vi "CloneClass.vi"(0 "ClassWriterGOOP300.lvclass":refnum<class "ClassWriterGOOP300.lvclass">, 1 "ClassRef":refnum<vi>, 2 "NewClassPath":path, 5 "error in (no error)":errorcluster) -> (14 "ClassWriterGOOP300.lvclass":refnum<class "ClassWriterGOOP300.lvclass">, 16 "NewClassPathOut(Might Be Modified)":path, 19 "error out":errorcluster)   [LabVIEW 2020, in "ClassWriterGOOP300.lvclass"]
uses:
  ClassWriterGOOP300.lvclass
  Provider_LvNativeClass/ClassWriterNative_class/ClassWriterNative.lvclass
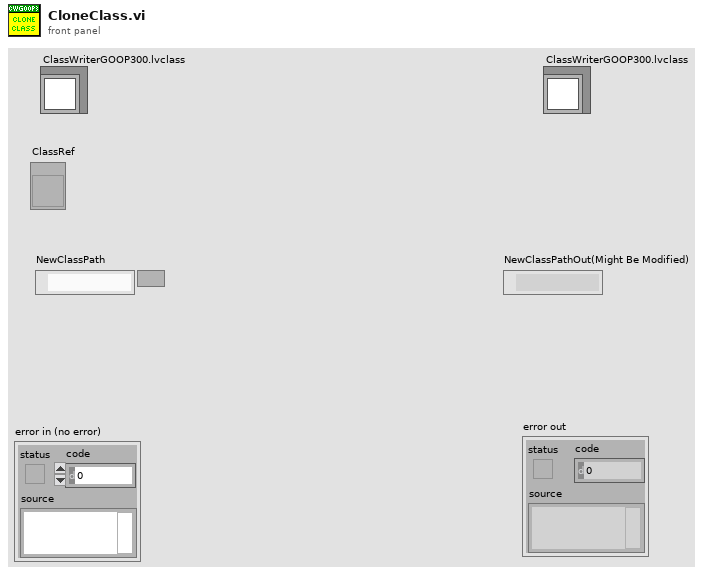
[diagram p1: front panel]
types:
  T1 = typedef "imagedata.ctl" = cluster{"image type":i32, "image depth":i32, "image":u8[], "mask":u8[], "colors":u32[], "Rectangle":cluster{"left":i16, "top":i16, "right":i16, "bottom":i16}}
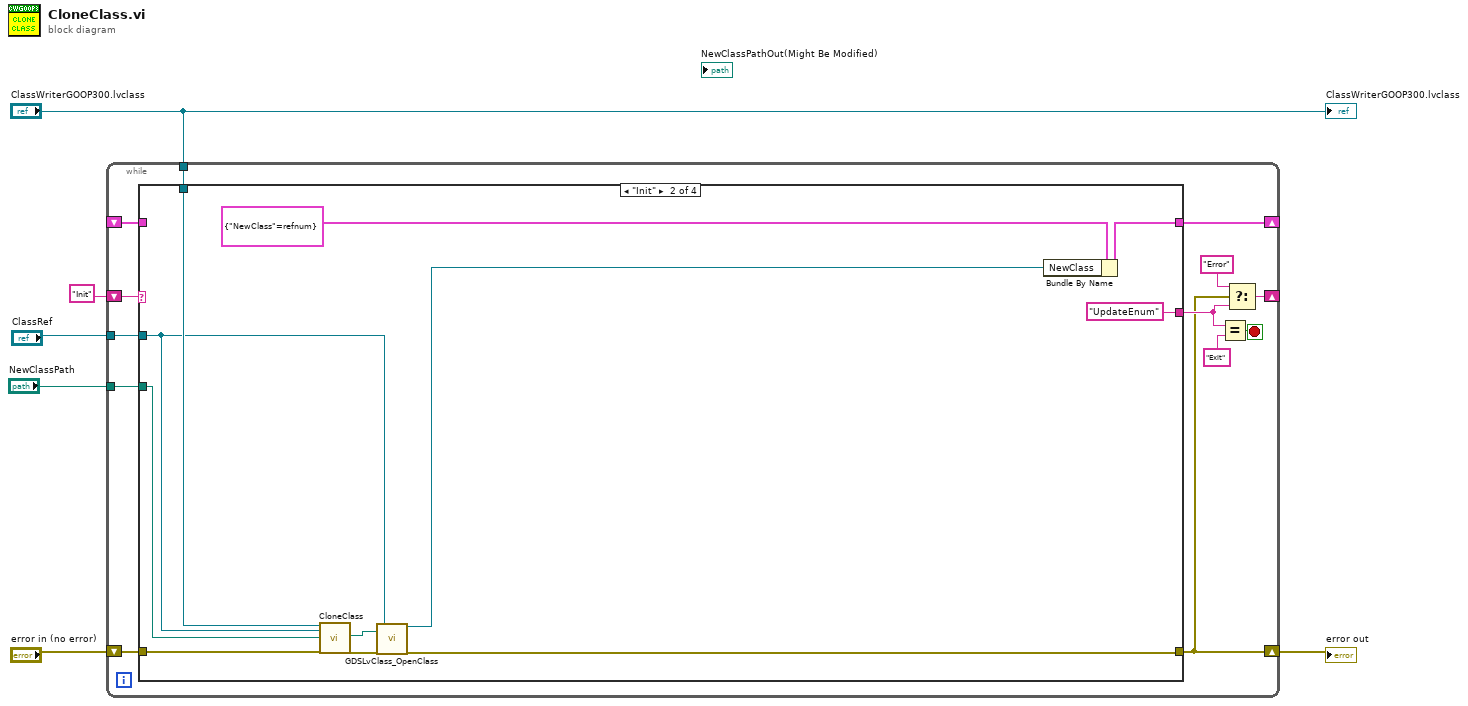
[diagram p0: block diagram]
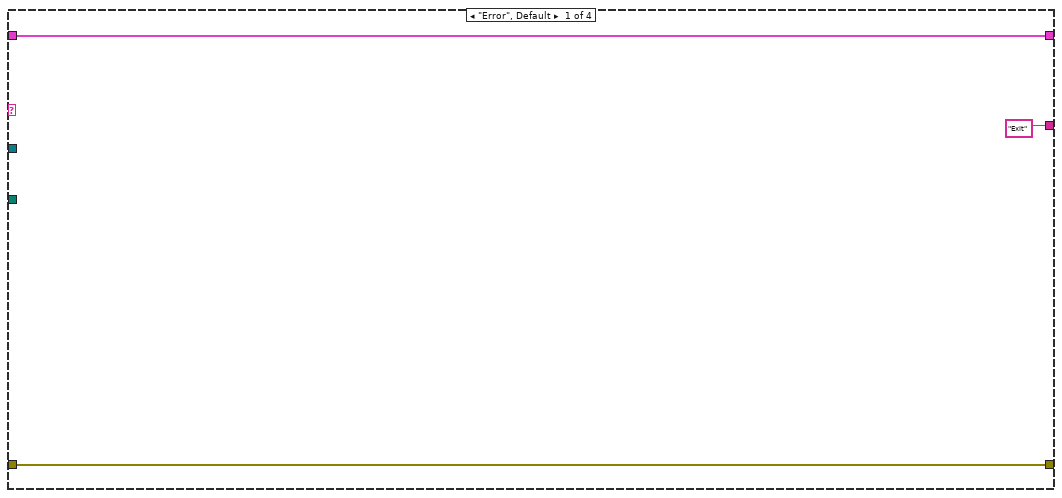
[diagram p2: hidden frame]
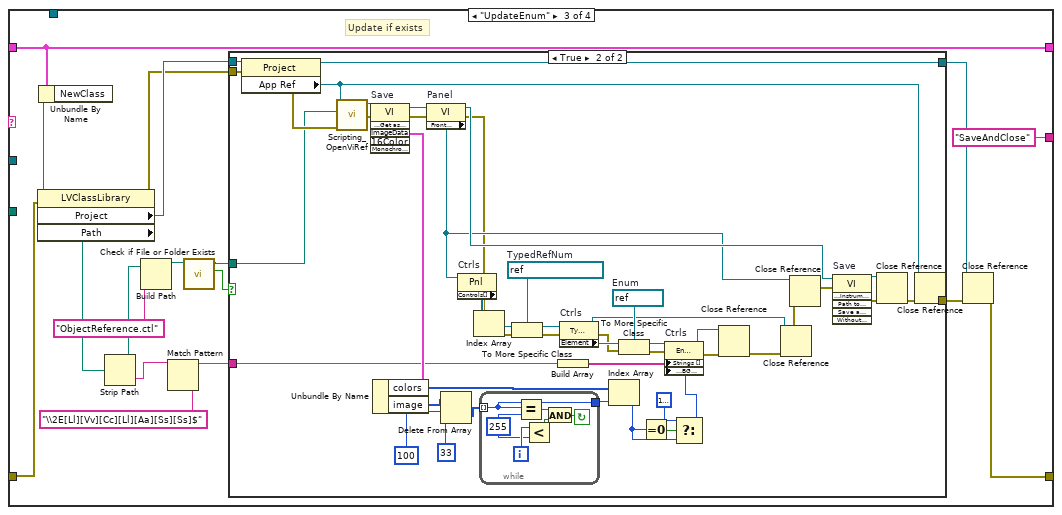
[diagram p3: hidden frame]
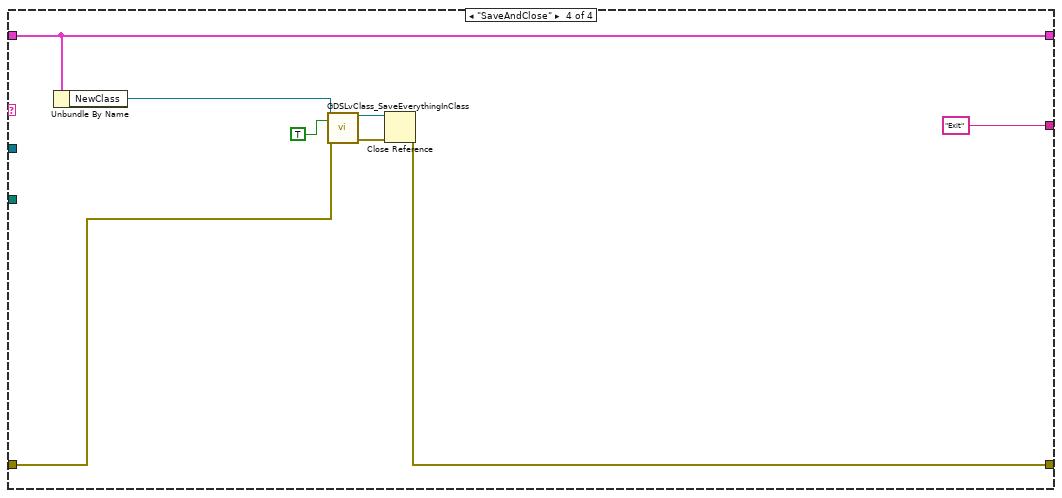
[diagram p5: hidden frame]
diagram:
  n1 = while {
    shift-right: [w12] -> w2
    shift-left: "error in (no error)" -> [w19]
    shift-right: [w17] -> _
    shift-left: "Init" -> [w18]
    shift-right: [w11] -> _
    shift-left: _ -> [w10]
    tunnel: "ClassWriterGOOP300.lvclass" -> [w9]
    tunnel: "ClassRef" -> [w8]
    tunnel: "NewClassPath" -> [w7]
    stop <- w16 stop-if-true
    n2 = case shown="\"Init\"" w18 {
      tunnel: w19 -> [w22 w30 w40 w108]
      tunnel: [w22 w26 w42 w111] -> w12
      tunnel: ["Exit" "UpdateEnum" "SaveAndClose" "Exit"] -> w13
      tunnel: [w20 w31 w50 w112] -> w11
      tunnel: w10 -> [w20 _ w50 w112]
      tunnel: w9 -> [_ w29 _ _]
      tunnel: w8 -> [_ w25 _ _]
      tunnel: w7 -> [_ w24 _ _]
      frame "Error", Default {
      }
      frame "Init" {
        n3 = call-parent "CloneClass.vi"("ClassWriterNative.lvclass"=w29, "ClassRef"=w25, "NewClassPath"=w24, "error in (no error)"=w30) -> ("NewClassPathOut(Might Be Modified)"=w23:path, "error out"=w28:errorcluster)  [unwired: 13 in, 1 out]
        n4 = call "GDSLvClass_OpenClass.vi"("ClassToOpen"=w23, "error in (no error)"=w28, "Project/ApplicationRef(If empty, currect active project will be used)"=w25) -> ("LVClass.Open"=w27:refnum<vi>, "error out"=w26:errorcluster)  [unwired: 15 in]
        n5 = Bundle By Name(cluster=cluster{"NewClass":refnum<vi>} {"NewClass"=refnum}, "NewClass"=w27) -> (w31:cluster{"NewClass":refnum<vi>})
      }
      frame "UpdateEnum" {
        # "Update if exists"
        n6 = Unbundle By Name(w50) -> ("NewClass"=w48:refnum<vi>)
        n7 = property class="LVClassLibrary"(reference=w48, error in=w40) -> (error out=w41:errorcluster, "Project"=w47:refnum<vi>, "Path"=w46:path)  [unwired: 1 out]
        n8 = Strip Path(path=w46) -> (stripped path=w45:path, name=w38:string)
        n9 = Build Path(base path=w45, name or relative path="ObjectReference.ctl") -> (appended path=w36:path)
        n10 = Match Pattern(string=w38, regular expression="\\2E[Ll][Vv][Cc][Ll][Aa][Ss][Ss]$") -> (before substring=w39:string)  [unwired: 1 in, 3 out]
        n11 = call <vilib>:"Check if File or Folder Exists.vi"("path"=w36) -> ("file or folder exists?"=w34:bool, "dup path"=w35:path)  [unwired: 8 in, 1 out]
        n12 = case shown="True" w34 {
          tunnel: w47 -> [w52 w59]
          tunnel: [w53 w58] -> w44
          tunnel: [w52 w57] -> w43
          tunnel: w41 -> [w53 w56]
          tunnel: w39 -> [_ w55]
          tunnel: w35 -> [_ w54]
          frame False {
          }
          frame True {
            w94 = refnum<vi> refnum  # Enum
            w97 = refnum<vi> refnum  # TypedRefNum
            n13 = property class="Project"(reference=w59, error in=w56) -> (reference out=w57:refnum<vi>, error out=w66:errorcluster, "App Ref"=w60:refnum<vi>)
            n14 = call "Scripting_OpenViRef.vi"("error in"=w66, "ViPath/ViName/Viref"=w54, "AppRef"=w60) -> ("error out"=w78:errorcluster, "vi reference"=w79:refnum<vi>)  [unwired: 6 in, 1 out]
            n15 = invoke on="Save" class="VI" method="VI Icon.Get as Image Data"(reference=w79, error in=w78) -> (reference out=w77:refnum<vi>, error out=w76:errorcluster, "ImageData"=w75:T1)  [unwired: 4 in, 3 out]
            n16 = Unbundle By Name(w75) -> ("colors"=w72:u32[], "image"=w74:u8[])
            n17 = property on="Panel" class="VI"(reference=w77, error in=w76) -> (reference out=w83:refnum<vi>, error out=w62:errorcluster, "Front Panel"=w63:refnum<vi>)
            n18 = Delete From Array(array=w74, length=100, index=33) -> (deleted portion=w65:u8[])  [unwired: 1 out]
            n19 = property on="Ctrls" class="Pnl"(reference=w63, error in=w62) -> ("Controls[]"=w99:refnum<vi>[])  [unwired: 2 out]
            n20 = Index Array(array=w99) -> (element=w98:refnum<vi>)  [unwired: 1 in]
            n21 = while {
              tunnel: w65 -> [w100] mode=indexing
              tunnel: [w100] -> w64
              i -> [w104]
              stop <- w101 continue-if-true
              w103 = 255
              n22 = Equal?(x=w100, y=w103) -> (x = y?=w105:bool)
              n23 = Less?(x=w104, y=w103) -> (x < y?=w102:bool)
              n24 = And(x=w105, y=w102) -> (x .and. y?=w101:bool)
            }
            n25 = To More Specific Class(target class=w97, reference=w98, error in=w62) -> (specific class reference=w96:refnum<vi>, error out=w91:errorcluster)
            n26 = Build Array(w55) -> (w92:string[])
            n27 = property on="Ctrls" class="TypRef"(reference=w96, error in=w91) -> (reference out=w85:refnum<vi>, error out=w90:errorcluster, "Element"=w95:refnum<vi>)
            n28 = Index Array(array=w72, index=w64) -> (element=w69:u32)
            n29 = To More Specific Class(target class=w94, reference=w95, error in=w90) -> (specific class reference=w93:refnum<vi>, error out=w89:errorcluster)
            n30 = Equal To 0?(x=w69) -> (x = 0?=w70:bool)
            n31 = Select(t=u32 16777216, s=w70, f=w69) -> (s? t:f=w68:u32)
            n32 = property on="Ctrls" class="Enum"(reference=w93, error in=w89, "Strings []"=w92, "Named Numeric Colors:BG Color"=w68) -> (reference out=w88:refnum<vi>, error out=w87:errorcluster)
            n33 = Close Reference(reference=w88, error in (no error)=w87) -> (error out=w86:errorcluster)
            n34 = Close Reference(reference=w85, error in (no error)=w86) -> (error out=w84:errorcluster)
            n35 = Close Reference(reference=w63, error in (no error)=w84) -> (error out=w82:errorcluster)
            n36 = invoke on="Save" class="VI" method="Save.Instrument"(reference=w83, error in=w82) -> (reference out=w81:refnum<vi>, error out=w80:errorcluster)  [unwired: 4 in, 4 out]
            n37 = Close Reference(reference=w81, error in (no error)=w80) -> (error out=w61:errorcluster)
            n38 = Close Reference(reference=w60, error in (no error)=w61) -> (error out=w58:errorcluster)
          }
        }
        n39 = Close Reference(reference=w43, error in (no error)=w44) -> (error out=w42:errorcluster)
      }
      frame "SaveAndClose" {
        n40 = Unbundle By Name(w112) -> ("NewClass"=w109:refnum<vi>)
        n41 = call "GDSLvClass_SaveEverythingInClass.vi"("ClassRefIn"=w109, "ForceResaving(False)"=TRUE, "error in"=w108) -> ("ClassRefOut"=w107:refnum<vi>, "error out"=w106:errorcluster)  [unwired: 15 in]
        n42 = Close Reference(reference=w107, error in (no error)=w106) -> (error out=w111:errorcluster)
      }
    }
    n43 = Equal?(x=w13, y="Exit") -> (x = y?=w16:bool)
    n44 = Select(t="Error", s=w12, f=w13) -> (s? t:f=w17:string)
  }
  "error out" <- w2
  "ClassWriterGOOP300.lvclass" <- "ClassWriterGOOP300.lvclass"
